vi "跑马灯组件.vi"(7 "error in (no error)":errorcluster caption="错误输入（无错误）") -> (0 "error out":errorcluster caption="错误输出", 3 "Lamp":bool[](array[boolean]))   [LabVIEW 2013]
uses:
  Step.ctl
  Status.ctl
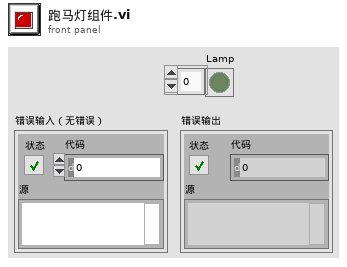
[diagram p1: front panel]
types:
  T1 = typedef "Step.ctl" = enum16{"Build Path", "Read Ini", "Run"}
  T2 = typedef "Status.ctl" = cluster{"Step":T1, "Ini Path":path, "Mode":u32[], "Timer":dbl[], "Length":i32, "Current Pos":i32}
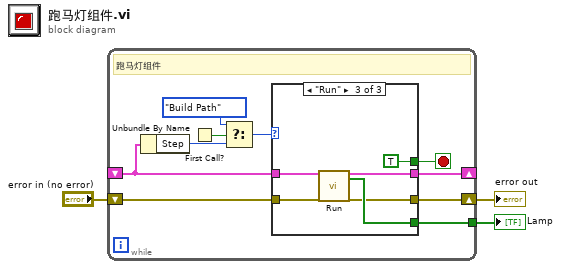
[diagram p0: block diagram]
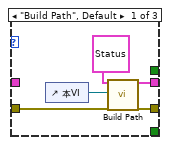
[diagram p2: hidden frame]
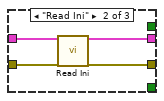
[diagram p3: hidden frame]
diagram:
  n1 = while {
    tunnel: [w10] -> w3
    shift-right: [w6] -> _
    shift-left: _ -> [w5]
    shift-right: [w7] -> w1
    shift-left: "error in (no error)" -> [w8]
    stop <- w9 stop-if-true
    # "跑马灯组件"
    n2 = Unbundle By Name(w5) -> ("Step"=w4:T1)
    n3 = First Call?() -> (First Call?: T/F=w13:bool)
    n4 = Select(t=Step."Build Path", s=w13, f=w4) -> (s? t:f=w12:T1)
    n5 = case shown="\"Run\"" w12 {
      tunnel: [_ _ w28] -> w10
      tunnel: [_ _ TRUE] -> w9
      tunnel: w8 -> [w18 w22 w26]
      tunnel: [w17 w21 w25] -> w7
      tunnel: [w14 w20 w24] -> w6
      tunnel: w5 -> [_ w19 w23]
      frame "Build Path", Default {
        n6 = control-ref of="本VI"() -> (w15:refnum<vi>)
        n7 = call "Build Path.vi"("Status输入"=T2 {"Step"=enum."Build Path", "Ini Path"=path "", "Mode"=[], "Timer"=[], "Length"=0, "Current Pos"=0} ("Status"), "VI输入"=w15, "错误输入（无错误）"=w18) -> ("Status输出"=w14:T2, "错误输出"=w17:errorcluster)  [unwired: 15 in]
      }
      frame "Read Ini" {
        n8 = call "Read Ini.vi"("Status输入"=w19, "错误输入（无错误）"=w22) -> ("Status输出"=w20:T2, "错误输出"=w21:errorcluster)  [unwired: 16 in]
      }
      frame "Run" {
        n9 = call "Run.vi"("Status输入"=w23, "错误输入（无错误）"=w26) -> ("Status输出"=w24:T2, "Lamp"=w28:bool[], "错误输出"=w25:errorcluster)  [unwired: 15 in]
      }
    }
  }
  "Lamp" <- w3
  "error out" <- w1
